vi "Add Points.vi"(7 "Num Array Out":i32[][](array[numeric]), 9 "Max Point":T1, 10 "Point Data":T2, 11 "Point":T1) -> (2 "Data Array Out":T2[](array[typedef]), 3 "Point Array Out":T1[](array[typedef]), 5 "Num Array Out 2":i32[][](array[numeric]))   [LabVIEW 2023]
uses:
  Cluster_Node.ctl
  Cluster_Point Data.ctl
  ENUM_Direction.ctl
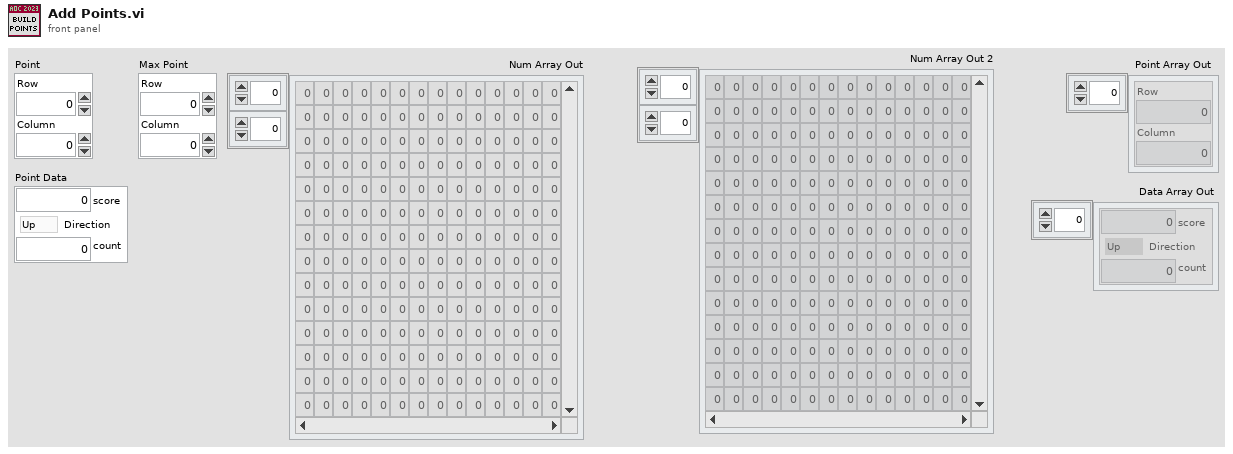
[diagram p1: front panel]
types:
  T1 = typedef "Cluster_Node.ctl" = cluster{"Row":i32, "Column":i32}
  T2 = typedef "Cluster_Point Data.ctl" = cluster{"score":i32, "Direction":T3, "count":i32}
  T3 = typedef "ENUM_Direction.ctl" = enum16{"Up", "Left", "Down", "Right"}
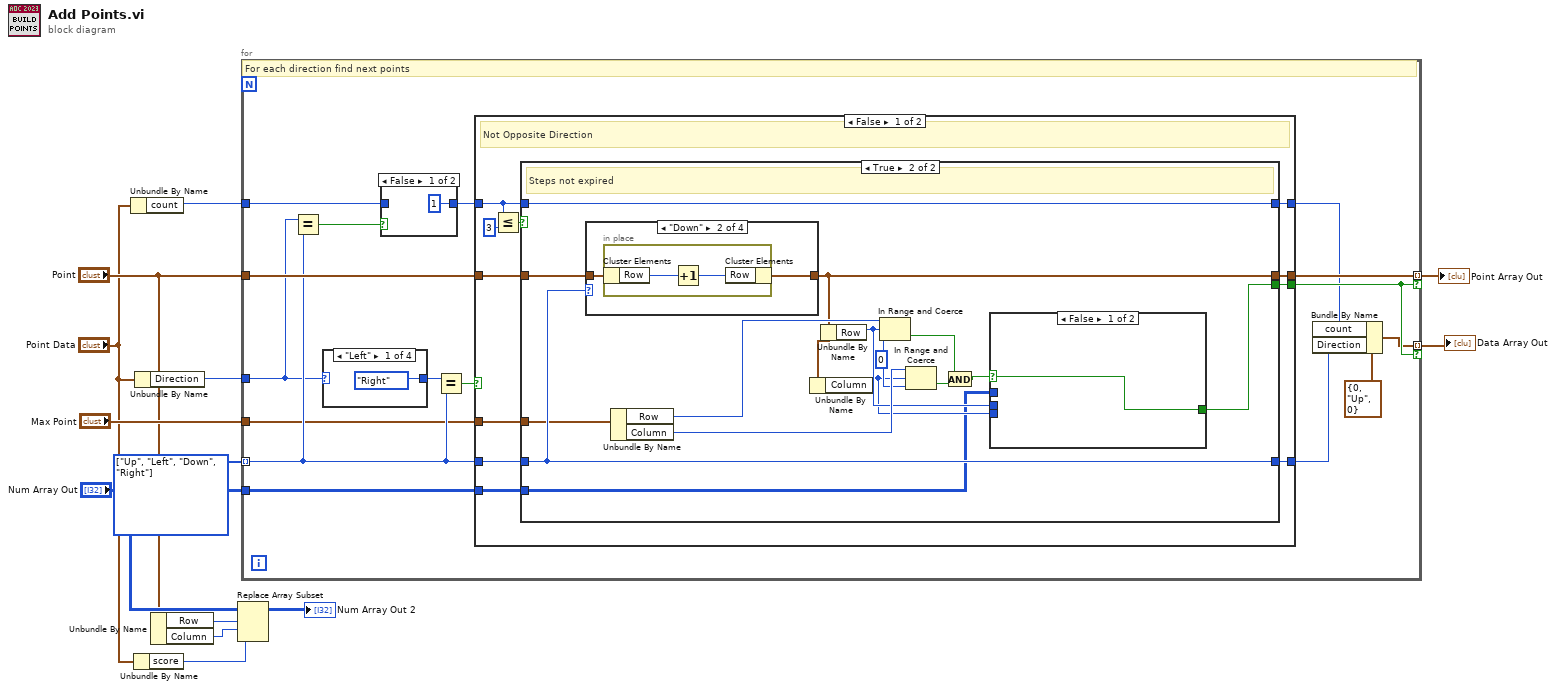
[diagram p0: block diagram]
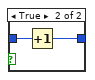
[diagram p2: hidden frame]
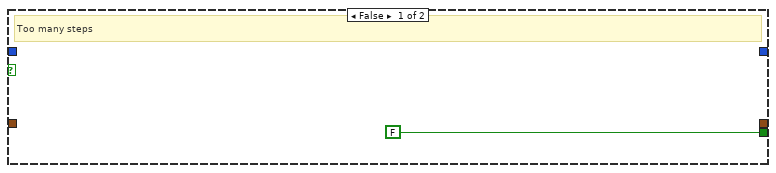
[diagram p3: hidden frame]
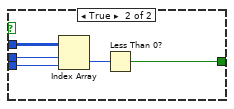
[diagram p4: hidden frame]
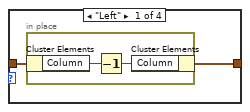
[diagram p5: hidden frame]
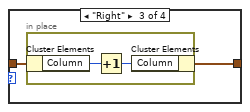
[diagram p6: hidden frame]
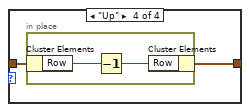
[diagram p7: hidden frame]
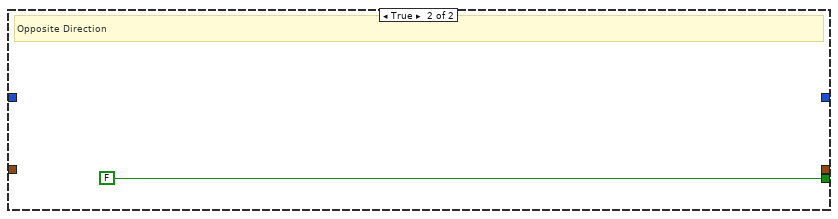
[diagram p8: hidden frame]
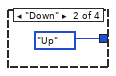
[diagram p9: hidden frame]
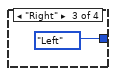
[diagram p10: hidden frame]
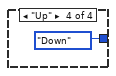
[diagram p11: hidden frame]
diagram:
  w13 = T3[] [enum."Up", enum."Left", enum."Down", enum."Right"] items=["Up", "Left", "Down", "Right"] ("Array")
  n1 = Unbundle By Name("Point Data") -> ("count"=w12:i32)
  n2 = Unbundle By Name("Point Data") -> ("score"=w1:i32)
  n3 = Unbundle By Name("Point Data") -> ("Direction"=w11:T3)
  n4 = Unbundle By Name("Point") -> ("Row"=w4:i32, "Column"=w3:i32)
  n5 = Replace Array Subset(array="Num Array Out", new element=w1, index (row)=w4, index (col)=w3) -> (→"Num Array Out 2":i32[][])
  n6 = for {
    tunnel: w13 -> [w26] mode=indexing
    tunnel: w11 -> [w25]
    tunnel: w12 -> [w24]
    tunnel: "Point" -> [w27]
    tunnel: [w21] -> w10 mode=indexing if=w20
    tunnel: [w18] -> w9 mode=indexing if=w20
    tunnel: "Max Point" -> [w15]
    tunnel: "Num Array Out" -> [w14]
    # "For each direction find next points"
    n7 = Equal?(x=w25, y=w26) -> (x = y?=w22:bool)
    n8 = case shown="\"Left\"" w25 {
      tunnel: [ENUM_Direction."Right" ("Direction") ENUM_Direction."Up" ("Direction") ENUM_Direction."Left" ("Direction") ENUM_Direction."Down" ("Direction")] -> w29
      frame "Left" {
      }
      frame "Down" {
      }
      frame "Right" {
      }
      frame "Up" {
      }
    }
    n9 = case shown="False" w22 {
      tunnel: w24 -> [_ w32]
      tunnel: [1 w31] -> w23
      frame False {
      }
      frame True {
        n10 = Increment(x=w32) -> (x+1=w31:i32)
      }
    }
    n11 = Equal?(x=w29, y=w26) -> (x = y?=w28:bool)
    n12 = case shown="False" w28 {
      tunnel: w26 -> [w43 _]
      tunnel: w27 -> [w39 _]
      tunnel: w23 -> [w40 _]
      tunnel: [w38 _] -> w21
      tunnel: [w37 FALSE] -> w20
      tunnel: [w36 _] -> w16
      tunnel: [w35 _] -> w17
      tunnel: w15 -> [w34 _]
      tunnel: w14 -> [w33 _]
      frame False {
        # "Not Opposite Direction"
        n13 = Less Or Equal?(x=w40, y=3) -> (x <= y?=w41:bool)
        n14 = case shown="True" w41 {
          tunnel: w43 -> [_ w57]
          tunnel: w40 -> [_ w58]
          tunnel: w39 -> [_ w59]
          tunnel: [_ w52] -> w38
          tunnel: [FALSE w45] -> w37
          tunnel: [_ w58] -> w36
          tunnel: [_ w57] -> w35
          tunnel: w34 -> [_ w56]
          tunnel: w33 -> [_ w46]
          frame False {
            # "Too many steps"
          }
          frame True {
            w53 = 0 ("lower limit")
            # "Steps not expired"
            n15 = case shown="\"Down\"" w57 {
              tunnel: w59 -> [w67 w71 w75 w79]
              tunnel: [w66 w70 w74 w78] -> w52
              frame "Left" {
                n16 = in-place {
                  n17 = in-place-cluster #1(w67) -> ("Column"=w69:i32)
                  n18 = Decrement(x=w69) -> (x-1=w68:i32)
                  n19 = in-place-cluster #1("Column"=w68) -> (w66:T1)
                }
              }
              frame "Down" {
                n20 = in-place {
                  n21 = in-place-cluster #2(w71) -> ("Row"=w73:i32)
                  n22 = Increment(x=w73) -> (x+1=w72:i32)
                  n23 = in-place-cluster #2("Row"=w72) -> (w70:T1)
                }
              }
              frame "Right" {
                n24 = in-place {
                  n25 = in-place-cluster #3(w75) -> ("Column"=w77:i32)
                  n26 = Increment(x=w77) -> (x+1=w76:i32)
                  n27 = in-place-cluster #3("Column"=w76) -> (w74:T1)
                }
              }
              frame "Up" {
                n28 = in-place {
                  n29 = in-place-cluster #4(w79) -> ("Row"=w81:i32)
                  n30 = Decrement(x=w81) -> (x-1=w80:i32)
                  n31 = in-place-cluster #4("Row"=w80) -> (w78:T1)
                }
              }
            }
            n32 = Unbundle By Name(w56) -> ("Row"=w55:i32, "Column"=w54:i32)
            n33 = Unbundle By Name(w52) -> ("Column"=w47:i32)
            n34 = Unbundle By Name(w52) -> ("Row"=w48:i32)
            n35 = In Range and Coerce(upper limit=w55, x=w48, lower limit=w53) -> (In Range?=w50:bool)  [unwired: 1 out]
            n36 = In Range and Coerce(upper limit=w54, x=w47, lower limit=w53) -> (In Range?=w51:bool)  [unwired: 1 out]
            n37 = And(x=w50, y=w51) -> (x .and. y?=w49:bool)
            n38 = case shown="False" w49 {
              selector: w49 -> [w60 _]
              tunnel: w46 -> [_ w65]
              tunnel: w48 -> [_ w64]
              tunnel: w47 -> [_ w63]
              tunnel: [w60 w61] -> w45
              frame False {
              }
              frame True {
                n39 = Index Array(array=w65, index (row)=w64, index (col)=w63) -> (element=w62:i32)
                n40 = Less Than 0?(x=w62) -> (x < 0?=w61:bool)
              }
            }
          }
        }
      }
      frame True {
        # "Opposite Direction"
      }
    }
    n41 = Bundle By Name(cluster=T2 {"score"=0, "Direction"=enum."Up", "count"=0} ("point Data"), "count"=w16, "Direction"=w17) -> (w18:T2)
  }
  "Point Array Out" <- w10
  "Data Array Out" <- w9
